vi "Write ERD Multiple Message Example.vi"(0 "GEA2 Reference In":refnum<k24>, 1 "Retry Count":u8=5, 2 "Read Timeout (ms)":u32=500, 5 "GEA Inputs":T3 {"Destination" format="%.0x"; "Source" format="%.0x"}, 7 "Write ERD List":T1[](array[typedef]) {"ERD Number" format="%.0x"}, 9 "Standalone?":bool=TRUE, 11 "Error In":errorcluster, 12 "#ERDs per message":i32=1 min=1 step=1, 13 "Verify ERD Response?":bool=TRUE) -> (4 "GEA2 Reference Out":refnum<k24>, 6 "Board ID":string, 8 "Raw Data Out":string[](array[string]), 15 "Error Out":errorcluster)   [LabVIEW 2016]
doc: "This is an example of how to use the GEA2 Write ERD multi-message VI. This VI splits up multiple ERD write requests into the number of messages you specify."
uses:
  Q:/Common/DLLs/GEA3/GeaCommunication.dll
  DLLs/GEA3/GeaCommunication.dll
  LabVIEW_GEA2_Toolkit.lvlibp/type defs/Source_Destination.ctl
  LabVIEW_GEA2_Toolkit.lvlibp/type defs/ERD Write Data In.ctl
  LabVIEW_GEA2_Toolkit.lvlibp/type defs/Data Type.ctl
  LabVIEW_GEA2_Toolkit.lvlibp
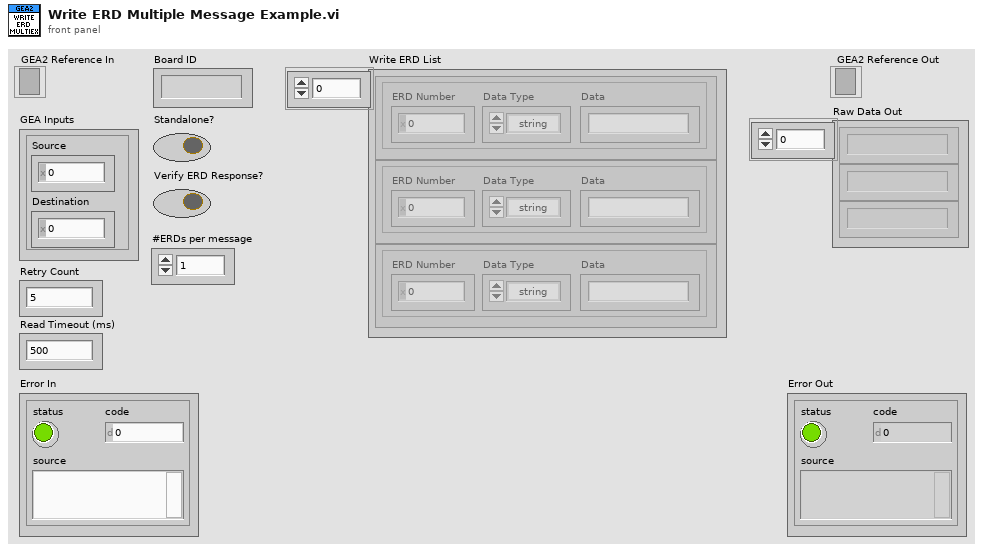
[diagram p1: front panel]
types:
  T1 = typedef "LabVIEW_GEA2_Toolkit.lvlibp/ERD Write Data In.ctl" = cluster{"ERD Number":u16, "Data Type":T2, "Data":string}
  T2 = typedef "LabVIEW_GEA2_Toolkit.lvlibp/Data Type.ctl" = enum16{"string", "boolean", "uint8_t", "uint16_t", "uint32_t", "uint64_t", "int8_t", "int16_t", "int32_t", "int64_t"}
  T3 = typedef "LabVIEW_GEA2_Toolkit.lvlibp/Source_Destination.ctl" = cluster{"Source":u8, "Destination":u8}
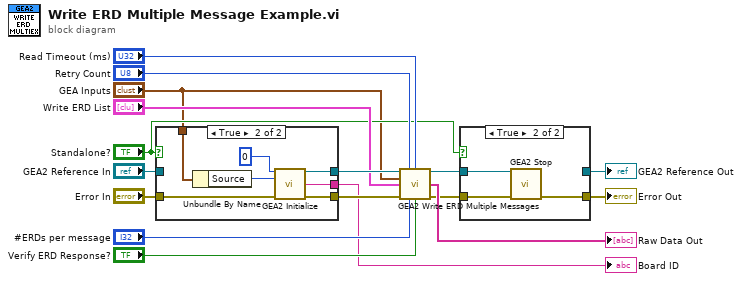
[diagram p0: block diagram]
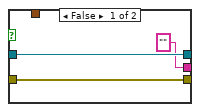
[diagram p3: hidden frame]
diagram:
  n1 = case shown="True" "Standalone?" {
    tunnel: [w19 w27] -> w14
    tunnel: "Error In" -> [w19 w26]
    tunnel: [w20 w24] -> w15
    tunnel: "GEA2 Reference In" -> [w20 _]
    tunnel: ["" ("Board ID") w23] -> w7
    tunnel: "GEA Inputs" -> [_ w22]
    frame False {
    }
    frame True {
      n2 = Unbundle By Name(w22) -> ("Source"=w21:u8)
      n3 = call "GEA2 Initialize.vi"("Board Index"=0, "Source Address"=w21, "error in"=w26) -> ("GEA2 Reference Out"=w24:refnum<k24>, "Board ID"=w23:string, "error out"=w27:errorcluster)  [unwired: 10 in]
    }
  }
  "Board ID" <- w7
  n4 = call "GEA2 Write ERD Multiple Messages.vi"("GEA2 Reference In"=w15, "# of Tries"="Retry Count", "Read Timeout (ms)"="Read Timeout (ms)", "GEA Inputs"="GEA Inputs", "Write ERD List"="Write ERD List", "Error In"=w14, "#ERDs per message"="#ERDs per message", "Verify ERD Response?"="Verify ERD Response?") -> ("GEA2 Reference Out"=w4:refnum<k24>, "Raw Data Out"=→"Raw Data Out":string[], "Error Out"=w5:errorcluster)  [unwired: 5 in]
  n5 = case shown="True" "Standalone?" {
    tunnel: [w29 w32] -> w6
    tunnel: w5 -> [w29 w31]
    tunnel: w4 -> [w28 w30]
    tunnel: [w28 _] -> w3
    frame False {
    }
    frame True {
      n6 = call "GEA2 Stop.vi"("GEA2 Reference In"=w30, "Error In"=w31) -> ("Error Out"=w32:errorcluster)  [unwired: 13 in]
    }
  }
  "Error Out" <- w6
  "GEA2 Reference Out" <- w3
